vi "img test13(calibration attempt1).vi"() -> ()   [LabVIEW 2014]
uses:
  <vilib>/vision/NI_Vision_Development_Module.lvlib
panel:
  out "bottom player 2":cluster{"Numeric":dbl, "Numeric":dbl}[](array[cluster])
  out "bottom player":cluster{"Numeric":dbl, "Numeric":dbl}[](array[cluster])
  out "top player":cluster{"Numeric":dbl, "Numeric":dbl}[](array[cluster])
  out "size(s)":i32
  in  "playing":bool
  out "Top VIew":cluster{"Numeric":dbl, "Numeric":dbl}[](graph)
  out "Image 4":T1(plugin-control)
  in  "frame jump":i32=3
  in  "speed":u32(slide)=200
  in  "start":i32(slide) step=219843704 scale=0.0..263.0
  out "Image 3":T1(plugin-control)
  out "Image 2":T1(plugin-control)
  in  "AVI Path":path=path "C:/Users/Kokum Weeratunga/Desktop/img processing/ChenJin vs HuYun.avi"
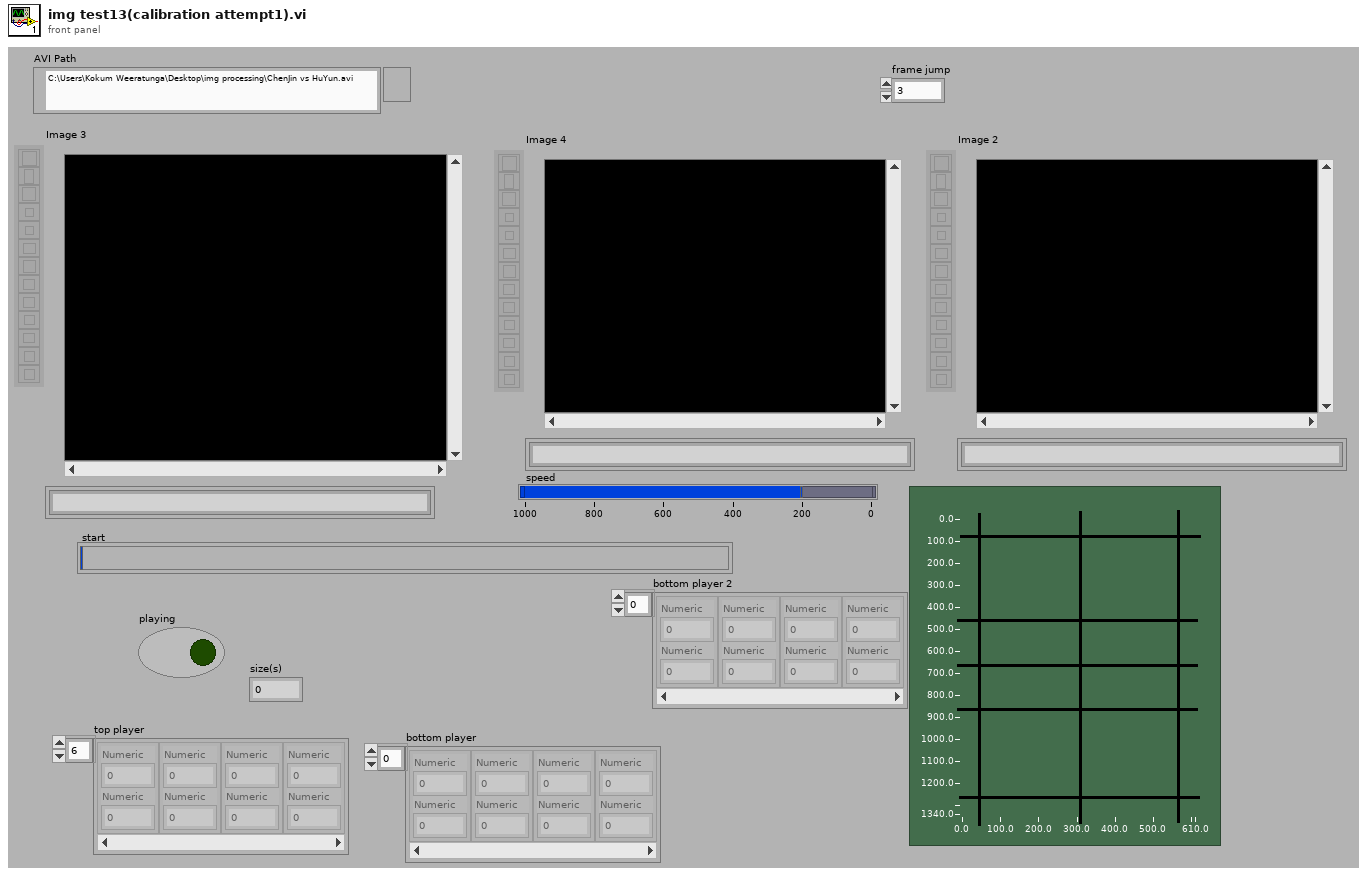
[diagram p1: front panel]
types:
  T1 = typedef "IMAQ Image.ctl" = refnum<image>
  T2 = typedef "Image Type" = u32
  T3 = typedef "AviRefnum.ctl" = refnum<k1>
  T4 = cluster{"width":u32, "height":u32, "framesPerSecond":u32, "compressionFilter":string, "hasData":bool}
  T5 = cluster{cluster{"X":sgl, "Y":sgl}[], cluster{i32, i32}[], "Unit":u32}
  T6 = cluster{"Origin Pixel":cluster{"X":sgl, "Y":sgl}, "Angle Relative to Horizontal (deg)":sgl, "Axis Reference":u32}
  T7 = typedef "Particle Parameters" = i32
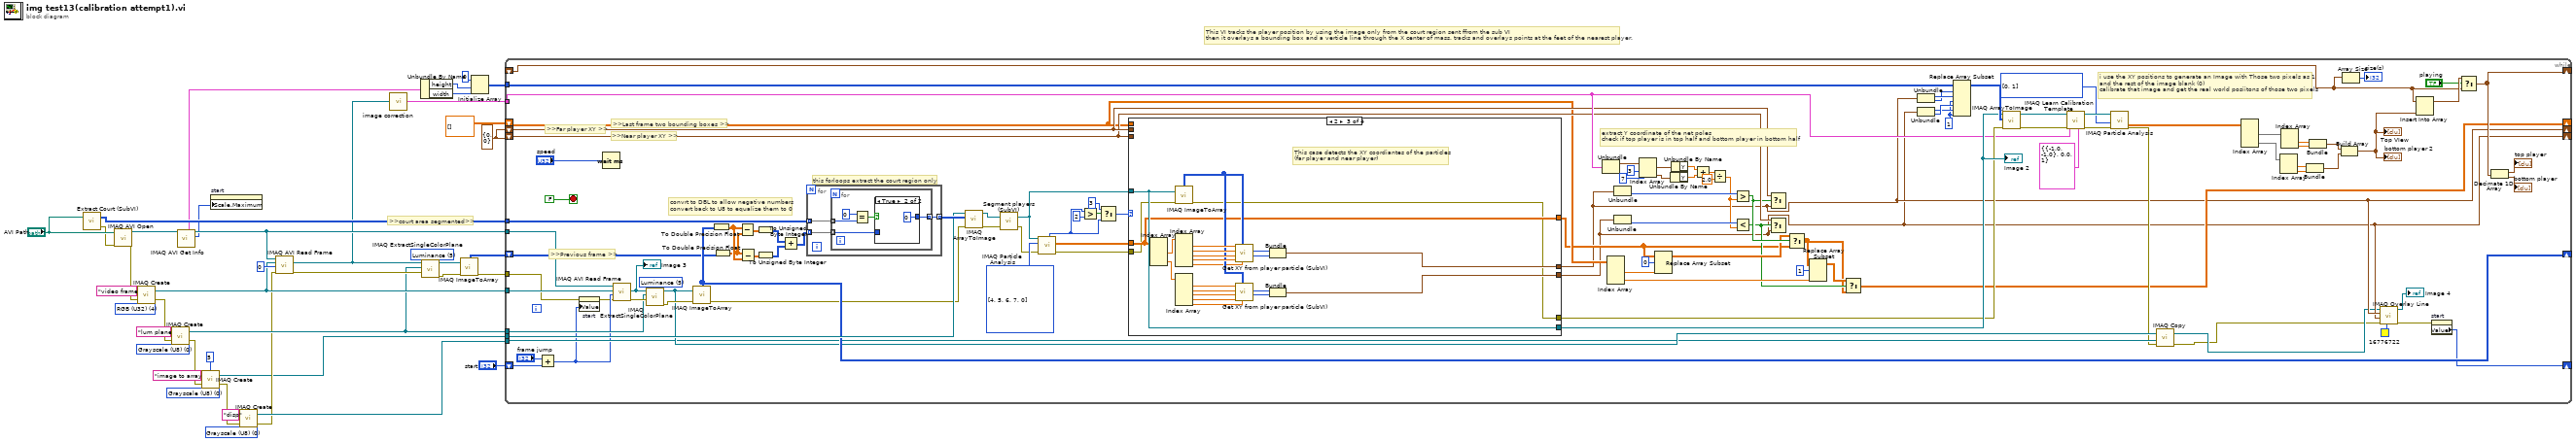
[diagram p0: block diagram]
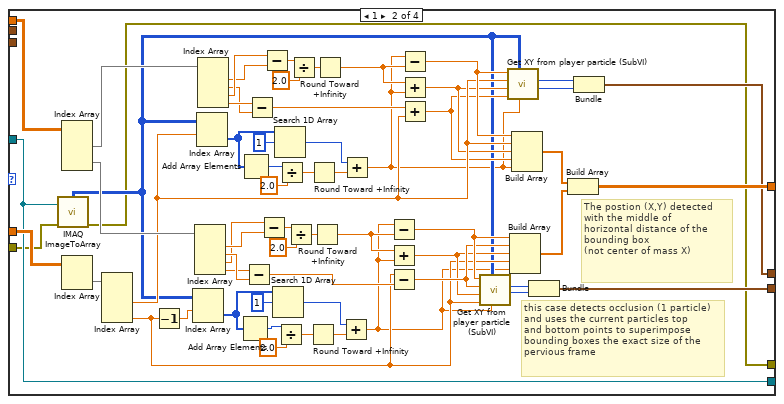
[diagram p3: hidden frame]
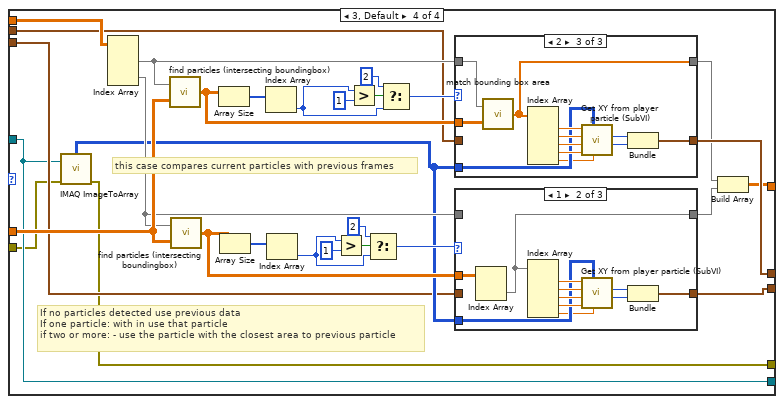
[diagram p4: hidden frame]
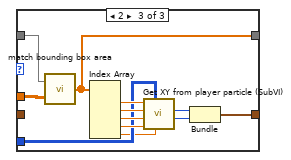
[diagram p6: hidden frame]
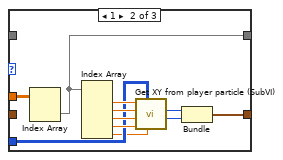
[diagram p8: hidden frame]
diagram:
  w13 = cluster{"X coordinate":i32, "Y coordinate":i32} {"X coordinate"=0, "Y coordinate"=0}
  w26 = T2 0 items=["Grayscale (U8)", "Grayscale (I16)", "Grayscale (SGL)", "Complex (CSG)", "RGB (U32)", "HSL (U32)", "RGB (U64)", "Grayscale (U16)"] ("Image Type")
  w33 = 5 items=["Red", "Green", "Blue", "Hue", "Saturation", "Luminance", "Value", "Intensity"] ("Color Plane")
  w34 = T2 0 items=["Grayscale (U8)", "Grayscale (I16)", "Grayscale (SGL)", "Complex (CSG)", "RGB (U32)", "HSL (U32)", "RGB (U64)", "Grayscale (U16)"] ("Image Type")
  w38 = T2 0 items=["Grayscale (U8)", "Grayscale (I16)", "Grayscale (SGL)", "Complex (CSG)", "RGB (U32)", "HSL (U32)", "RGB (U64)", "Grayscale (U16)"] ("Image Type")
  w36 = T2 4 items=["Grayscale (U8)", "Grayscale (I16)", "Grayscale (SGL)", "Complex (CSG)", "RGB (U32)", "HSL (U32)", "RGB (U64)", "Grayscale (U16)"] ("Image Type")
  # ">>court area segmented>>"
  # "This VI tracks the player position by using the image only from the court region sent ffrom the sub VI\nthen it overlays a bounding box and a verticle line through the X center of mass. tracks and overlays points at the feet of the nearest player."
  n1 = call "Extract Court (SubVI).vi"("AVI Path"="AVI Path") -> ("error out"=w40:errorcluster, "Court pixels out"=w16:u8[][])  [unwired: 1 in]
  n2 = call "IMAQ AVI Open"("error in (no error)"=w40, "AVI Path"="AVI Path") -> ("error out"=w22:errorcluster, "Avi Refnum"=w11:T3)  [unwired: 8 in]
  n3 = call "IMAQ Create"("Image Name"="video frame", "Image Type"=w36, "error in (no error)"=w22) -> ("New Image"=w30:T1, "error out"=w21:errorcluster)  [unwired: 2 in]
  n4 = call "IMAQ Create"("Image Name"="lum plane", "Image Type"=w38, "error in (no error)"=w21) -> ("New Image"=w29:T1, "error out"=w20:errorcluster)  [unwired: 2 in]
  n5 = call "IMAQ AVI Get Info"("Avi Refnum"=w11) -> ("Number of Frames"=w9:u32, "Avi Refnum (duplicate)"=w10:T3, "Frame Data"=w6:T4)  [unwired: 6 in, 2 out]
  n6 = call "IMAQ Create"("Border Size"=5, "Image Name"="image to array", "Image Type"=w34, "error in (no error)"=w20) -> ("New Image"=w15:T1, "error out"=w19:errorcluster)  [unwired: 1 in]
  n7 = property on="start" class="Slide (strict)"("Scale.Maximum"=w9) -> ()  [unwired: 2 in, 2 out]
  n8 = call "IMAQ Create"("Image Name"="disp", "Image Type"=w26, "error in (no error)"=w19) -> ("New Image"=w24:T1, "error out"=w18:errorcluster)  [unwired: 2 in]
  n9 = call "IMAQ AVI Read Frame"("error in (no error)"=w18, "Frame Number"=u32 0, "Image"=w30, "Avi Refnum"=w10) -> ("error out"=w32:errorcluster, "Image Out"=w2:T1)  [unwired: 4 in, 2 out]
  n10 = call "image correction.vi"("Image"=w2) -> ("ref points"=w1:T5)
  n11 = Unbundle By Name(w6) -> ("height"=w5:u32, "width"=w4:u32)
  n12 = call "IMAQ ExtractSingleColorPlane"("Color Plane"=w33, "error in (no error)"=w32, "Image Dst"=w29, "Image Src"=w2) -> ("error out"=w23:errorcluster, "Image Dst Out"=w27:T1)  [unwired: 6 in]
  n13 = call "IMAQ ImageToArray"("error in (no error)"=w23, "Image"=w27) -> ("error out"=w8:errorcluster, "Image Pixels (U8)"=w28:u8[][])  [unwired: 2 in, 3 out]
  n14 = Initialize Array(u8 0 ("element"), w5, w4) -> (w3:u8[][])
  n15 = while {
    tunnel: w10 -> [w111]
    tunnel: w30 -> [w131]
    tunnel: w16 -> [w148]
    tunnel: w29 -> [w132]
    tunnel: w15 -> [w145]
    shift-right: [w144] -> _
    shift-left: w28 -> [w143]
    tunnel: w24 -> [w114]
    shift-right: [w48] -> _
    shift-left: dbl[][] [] ("Particle Measurements (Pixels)") -> [w58]
    shift-right: [w46] -> _
    shift-left: w13 -> [w60]
    shift-right: [w45] -> _
    shift-left: w13 -> [w59]
    shift-right: [w106] -> _
    shift-left: "start" -> [w113]
    tunnel: w8 -> [w109]
    tunnel: w3 -> [w105]
    tunnel: w1 -> [w73]
    shift-right: [w76] -> _
    shift-left: _ -> [w80]
    stop <- FALSE stop-if-true
    w91 = T7[] [0, 1] items=["Center of Mass X", "Center of Mass Y", "First Pixel X", "First Pixel Y", "Bounding Rect Left", "Bounding Rect Top", "Bounding Rect Right", "Bounding Rect Bottom", "Max Feret Diameter Start X", "Max Feret Diameter Start Y", "Max Feret Diameter End X", "Max Feret Diameter End Y", "Max Horiz. Segment Length Left", "Max Horiz. Segment Length Right", "Max Horiz. Segment Length Row", "-", "Bounding Rect Width", "Bounding Rect Height", "Bounding Rect Diagonal", "Perimeter", "Convex Hull Perimeter", "Holes' Perimeter", "Max Feret Diameter", "Equivalent Ellipse Major Axis", "Equivalent Ellipse Minor Axis", "Equivalent Ellipse Minor Axis (Feret)", "Equivalent Rect Long Side", "Equivalent Rect Short Side", "Equivalent Rect Diagonal", "Equivalent Rect Short Side (Feret)", "Average Horiz. Segment Length", "Average Vert. Segment Length", "Hydraulic Radius", "Waddel Disk Diameter", "-", "Area", "Holes' Area", "Particle & Holes' Area", "Convex Hull Area", "Image Area", "-", "Number of Holes", "Number of Horiz. Segments", "Number of Vert. Segments", "-", "Orientation", "Max Feret Diameter Orientation", "-", "% Area/Image Area", "% Area/(Particle & Holes' Area)", "Ratio of Equivalent Ellipse Axes", "Ratio of Equivalent Rect Sides", "-", "Elongation Factor", "Compactness Factor", "Heywood Circularity Factor", "Type Factor", "-", "Sum X", "Sum Y", "Sum XX", "Sum XY", "Sum YY", "Sum XXX", "Sum XXY", "Sum XYY", "Sum YYY", "-", "Moment of Inertia XX", "Moment of Inertia XY", "Moment of Inertia YY", "Moment of Inertia XXX", "Moment of Inertia XXY", "Moment of Inertia XYY", "Moment of Inertia YYY", "Norm. Moment of Inertia XX", "Norm. Moment of Inertia XY", "Norm. Moment of Inertia YY", "Norm. Moment of Inertia XXX", "Norm. Moment of Inertia XXY", "Norm. Moment of Inertia XYY", "Norm. Moment of Inertia YYY", "Hu Moment 1", "Hu Moment 2", "Hu Moment 3", "Hu Moment 4", "Hu Moment 5", "Hu Moment 6", "Hu Moment 7"] ("Real-World Measurements")
    w100 = u8 1 ("new element/subarray")
    w133 = T7[] [4, 5, 6, 7, 0] items=["Center of Mass X", "Center of Mass Y", "First Pixel X", "First Pixel Y", "Bounding Rect Left", "Bounding Rect Top", "Bounding Rect Right", "Bounding Rect Bottom", "Max Feret Diameter Start X", "Max Feret Diameter Start Y", "Max Feret Diameter End X", "Max Feret Diameter End Y", "Max Horiz. Segment Length Left", "Max Horiz. Segment Length Right", "Max Horiz. Segment Length Row", "-", "Bounding Rect Width", "Bounding Rect Height", "Bounding Rect Diagonal", "Perimeter", "Convex Hull Perimeter", "Holes' Perimeter", "Max Feret Diameter", "Equivalent Ellipse Major Axis", "Equivalent Ellipse Minor Axis", "Equivalent Ellipse Minor Axis (Feret)", "Equivalent Rect Long Side", "Equivalent Rect Short Side", "Equivalent Rect Diagonal", "Equivalent Rect Short Side (Feret)", "Average Horiz. Segment Length", "Average Vert. Segment Length", "Hydraulic Radius", "Waddel Disk Diameter", "-", "Area", "Holes' Area", "Particle & Holes' Area", "Convex Hull Area", "Image Area", "-", "Number of Holes", "Number of Horiz. Segments", "Number of Vert. Segments", "-", "Orientation", "Max Feret Diameter Orientation", "-", "% Area/Image Area", "% Area/(Particle & Holes' Area)", "Ratio of Equivalent Ellipse Axes", "Ratio of Equivalent Rect Sides", "-", "Elongation Factor", "Compactness Factor", "Heywood Circularity Factor", "Type Factor", "-", "Sum X", "Sum Y", "Sum XX", "Sum XY", "Sum YY", "Sum XXX", "Sum XXY", "Sum XYY", "Sum YYY", "-", "Moment of Inertia XX", "Moment of Inertia XY", "Moment of Inertia YY", "Moment of Inertia XXX", "Moment of Inertia XXY", "Moment of Inertia XYY", "Moment of Inertia YYY", "Norm. Moment of Inertia XX", "Norm. Moment of Inertia XY", "Norm. Moment of Inertia YY", "Norm. Moment of Inertia XXX", "Norm. Moment of Inertia XXY", "Norm. Moment of Inertia XYY", "Norm. Moment of Inertia YYY", "Hu Moment 1", "Hu Moment 2", "Hu Moment 3", "Hu Moment 4", "Hu Moment 5", "Hu Moment 6", "Hu Moment 7"] ("Pixel Measurements")
    w149 = 5 items=["Red", "Green", "Blue", "Hue", "Saturation", "Luminance", "Value", "Intensity"] ("Color Plane")
    # "extract Y coordinate of the net poles\ncheck if top player is in top half and bottom player in bottom half"
    # "i use the XY positions to generate an Image with Those two pixels as 1 \nand the rest of the image blank (0)\ncalibrate that image and get the real world posiitons of those two pixels"
    # ">>Last frame two bounding boxes >>"
    # ">>Far player XY >>"
    # ">>Near player XY >>"
    # ">>Previous frame >>"
    # "convrt to DBL to allow negative numbers\nconvert back to U8 to equalize them to 0"
    # "this forloops extract the court region only"
    n16 = Add(x="frame jump", y=w113) -> (x+y=w110:i32)
    n17 = property on="start" class="Slide (strict)"(error in=w109, "Value"=w110) -> (error out=w108:errorcluster)  [unwired: 1 in, 1 out]
    n18 = Wait (ms)(milliseconds to wait="speed") -> ()  [unwired: 1 out]
    n19 = call "IMAQ AVI Read Frame"("error in (no error)"=w108, "Frame Number"=w110, "Image"=w131, "Avi Refnum"=w111) -> ("error out"=w150:errorcluster, "Image Out"=w128:T1)  [unwired: 4 in, 2 out]
    "Image 3" <- w128
    n20 = call "IMAQ ExtractSingleColorPlane"("Color Plane"=w149, "error in (no error)"=w150, "Image Dst"=w132, "Image Src"=w128) -> ("error out"=w135:errorcluster, "Image Dst Out"=w115:T1)  [unwired: 6 in]
    n21 = call "IMAQ ImageToArray"("error in (no error)"=w135, "Image"=w115) -> ("error out"=w134:errorcluster, "Image Pixels (U8)"=w144:u8[][])  [unwired: 2 in, 3 out]
    n22 = To Double Precision Float(number=w144) -> (double precision float=w139:dbl[][])
    n23 = To Double Precision Float(number=w143) -> (double precision float=w138:dbl[][])
    n24 = Subtract(x=w139, y=w138) -> (x-y=w137:dbl[][])
    n25 = Subtract(x=w138, y=w139) -> (x-y=w136:dbl[][])
    n26 = To Unsigned Byte Integer(number=w137) -> (unsigned 8bit integer=w142:u8[][])
    n27 = To Unsigned Byte Integer(number=w136) -> (unsigned 8bit integer=w141:u8[][])
    n28 = Add(x=w142, y=w141) -> (x+y=w140:u8[][])
    n29 = for {
      tunnel: w148 -> [w321] mode=indexing
      tunnel: [w320] -> w146 mode=indexing
      tunnel: w140 -> [w319] mode=indexing
      n30 = for {
        tunnel: w321 -> [w326] mode=indexing
        tunnel: [w323] -> w320 mode=indexing
        tunnel: w319 -> [w322] mode=indexing
        n31 = Equal?(x=u8 0, y=w326) -> (x = y?=w324:bool)
        n32 = case shown="True" w324 {
          tunnel: [w327 u8 0 ("x")] -> w323
          tunnel: w322 -> [w327 _]
          frame False {
          }
          frame True {
          }
        }
      }
    }
    n33 = call "IMAQ ArrayToImage"("error in (no error)"=w134, "Image Pixels (U8)"=w146, "Image"=w145) -> ("error out"=w129:errorcluster, "Image Out"=w130:T1)  [unwired: 7 in]
    n34 = call "Segment players (SubVI).vi"("error In"=w129, "Image In"=w130) -> ("error out"=w122:errorcluster, "Image Out"=w120:T1)
    n35 = call "IMAQ Particle Analysis"("error in (no error)"=w122, "Pixel Measurements"=w133, "Image"=w120) -> ("error out"=w121:errorcluster, "Particle Measurements (Pixels)"=w119:dbl[][], "Number of Particles"=w124:i32)  [unwired: 3 in, 3 out]
    n36 = Greater?(x=w124, y=2) -> (0:w127:bool)
    n37 = Select(t=3 ("y"), s=w127, f=w124) -> (s? t:f=w123:i32)
    n38 = case shown="2" w123 {
      tunnel: [w154 w181 w235 w245] -> w98
      tunnel: w119 -> [_ w216 w223 w265]
      tunnel: w121 -> [w151 w157 w220 w241]
      tunnel: w120 -> [w154 w181 w235 w245]
      tunnel: [w152 w165 w225 w247] -> w45
      tunnel: [w153 w172 w224 w246] -> w46
      tunnel: [w155 w182 w223 w242] -> w47
      tunnel: w58 -> [w155 w206 _ w268]
      tunnel: w60 -> [w153 _ _ w253]
      tunnel: w59 -> [w152 _ _ w248]
      tunnel: [w151 w156 w219 w240] -> w97
      frame 0 {
        # "This case identifies frames where no particles are detected and keeps the same values from the\nprevious frame"
      }
      frame 1 {
        # "The postion (X,Y) detected with the middle of \nhorizontal distance of the bounding box\n(not center of mass X)"
        # "this case detects occlusion (1 particle)\nand uses the current particles top \nand bottom points to superimpose \nbounding boxes the exact size of the \npervious frame"
        n39 = call "IMAQ ImageToArray"("error in (no error)"=w157, "Image"=w181) -> ("error out"=w156:errorcluster, "Image Pixels (U8)"=w164:u8[][])  [unwired: 2 in, 3 out]
        n40 = Index Array(array=w206) -> (element #1=w214:dbl[], element #2=w186:dbl[])  [unwired: 4 in]
        n41 = Index Array(array=w216) -> (element=w215:dbl[])  [unwired: 2 in]
        n42 = Index Array(array=w215) -> (element #2=w177:dbl, element #4=w168:dbl)  [unwired: 4 in, 2 out]
        n43 = Decrement(x=w168) -> (x-1=w179:dbl)
        n44 = Index Array(array=w164, index (row)=w179) -> (element=w201:u8[])  [unwired: 1 in]
        n45 = Index Array(array=w186) -> (element #1=w190:dbl, element #2=w193:dbl, element #3=w189:dbl, element #4=w192:dbl)  [unwired: 4 in]
        n46 = Index Array(array=w164, index (row)=w177) -> (element=w194:u8[])  [unwired: 1 in]
        n47 = Index Array(array=w214) -> (element #1=w210:dbl, element #2=w207:dbl, element #3=w211:dbl, element #4=w208:dbl)  [unwired: 4 in]
        n48 = Add Array Elements(numeric array=w201) -> (sum=w202:u8)
        n49 = Add Array Elements(numeric array=w194) -> (sum=w198:u8)
        n50 = Subtract(x=w192, y=w193) -> (x-y=w180:dbl)
        n51 = Subtract(x=w208, y=w207) -> (x-y=w185:dbl)
        n52 = Subtract(x=w189, y=w190) -> (x-y=w188:dbl)
        n53 = Subtract(x=w211, y=w210) -> (x-y=w212:dbl)
        n54 = Search 1D Array(1D array=w201, element=u8 1) -> (index of element=w200:i32)  [unwired: 1 in]
        n55 = Search 1D Array(1D array=w194, element=u8 1) -> (index of element=w199:i32)  [unwired: 1 in]
        n56 = Divide(x=w202, y=2.0) -> (x/y=w203:dbl)
        n57 = Divide(x=w198, y=2.0) -> (x/y=w197:dbl)
        n58 = Divide(x=w188, y=2.0) -> (x/y=w191:dbl)
        n59 = Divide(x=w212, y=2.0) -> (x/y=w209:dbl)
        n60 = Round Toward +Infinity(x=w203) -> (ceil(x): smallest int >= x=w162:dbl)
        n61 = Round Toward +Infinity(x=w197) -> (ceil(x): smallest int >= x=w161:dbl)
        n62 = Round Toward +Infinity(x=w191) -> (ceil(x): smallest int >= x=w163:dbl)
        n63 = Round Toward +Infinity(x=w209) -> (ceil(x): smallest int >= x=w160:dbl)
        n64 = Add(x=w200, y=w162) -> (x+y=w158:dbl)
        n65 = Add(x=w199, y=w161) -> (x+y=w159:dbl)
        n66 = Subtract(x=w158, y=w163) -> (x-y=w171:dbl)
        n67 = Add(x=w163, y=w158) -> (x+y=w169:dbl)
        n68 = Subtract(x=w168, y=w180) -> (x-y=w170:dbl)
        n69 = Subtract(x=w159, y=w160) -> (x-y=w178:dbl)
        n70 = Add(x=w160, y=w159) -> (x+y=w176:dbl)
        n71 = Add(x=w185, y=w177) -> (x+y=w175:dbl)
        n72 = call "Get XY from player particle (SubVI).vi"("Center of mass X"=w158, "Image in Pixels (U8)"=w164, "Particle bounding rect bottom"=w168, "Particle bounding rect right"=w169, "Particle bounding rect top"=w170, "Particle bounding rect left"=w171) -> ("Y coordinate"=w166:i32, "X coordinate"=w167:i32)  [unwired: 1 in, 1 out]
        n73 = call "Get XY from player particle (SubVI).vi"("Center of mass X"=w159, "Image in Pixels (U8)"=w164, "Particle bounding rect bottom"=w175, "Particle bounding rect right"=w176, "Particle bounding rect top"=w177, "Particle bounding rect left"=w178) -> ("Y coordinate"=w173:i32, "X coordinate"=w174:i32)  [unwired: 1 in, 1 out]
        n74 = Build Array(w171, w170, w169, w168, w158) -> (w183:dbl[])
        n75 = Build Array(w178, w177, w176, w175, w159) -> (w184:dbl[])
        n76 = Bundle("X coordinate"=w167, "Y coordinate"=w166) -> (w165:cluster{"X coordinate":i32, "Y coordinate":i32})  [unwired: 1 in]
        n77 = Build Array(w184, w183) -> (w182:dbl[][])
        n78 = Bundle("X coordinate"=w174, "Y coordinate"=w173) -> (w172:cluster{"X coordinate":i32, "Y coordinate":i32})  [unwired: 1 in]
      }
      frame 2 {
        # "This case detects the XY coordiantes of the particles\n(far player and near player)"
        n79 = Index Array(array=w223) -> (element #1=w229:dbl[], element #2=w228:dbl[])  [unwired: 4 in]
        n80 = call "IMAQ ImageToArray"("error in (no error)"=w220, "Image"=w235) -> ("error out"=w219:errorcluster, "Image Pixels (U8)"=w230:u8[][])  [unwired: 2 in, 3 out]
        n81 = Index Array(array=w229) -> (element #1=w239:dbl, element #2=w238:dbl, element #3=w237:dbl, element #4=w236:dbl, element #5=w222:dbl)  [unwired: 5 in]
        n82 = Index Array(array=w228) -> (element #1=w231:dbl, element #2=w232:dbl, element #3=w233:dbl, element #4=w234:dbl, element #5=w221:dbl)  [unwired: 5 in]
        n83 = call "Get XY from player particle (SubVI).vi"("Center of mass X"=w222, "Image in Pixels (U8)"=w230, "Particle bounding rect bottom"=w236, "Particle bounding rect right"=w237, "Particle bounding rect top"=w238, "Particle bounding rect left"=w239) -> ("Y coordinate"=w218:i32, "X coordinate"=w227:i32)  [unwired: 1 in, 1 out]
        n84 = call "Get XY from player particle (SubVI).vi"("Center of mass X"=w221, "Image in Pixels (U8)"=w230, "Particle bounding rect bottom"=w234, "Particle bounding rect right"=w233, "Particle bounding rect top"=w232, "Particle bounding rect left"=w231) -> ("Y coordinate"=w217:i32, "X coordinate"=w226:i32)  [unwired: 1 in, 1 out]
        n85 = Bundle("X coordinate"=w227, "Y coordinate"=w218) -> (w224:cluster{"X coordinate":i32, "Y coordinate":i32})  [unwired: 1 in]
        n86 = Bundle("X coordinate"=w226, "Y coordinate"=w217) -> (w225:cluster{"X coordinate":i32, "Y coordinate":i32})  [unwired: 1 in]
      }
      frame 3, Default {
        # "If no particles detected use previous data\nIf one particle: with in use that particle\nif two or more: - use the particle with the closest area to previous particle"
        # "this case compares current particles with previous frames"
        n87 = call "IMAQ ImageToArray"("error in (no error)"=w241, "Image"=w245) -> ("error out"=w240:errorcluster, "Image Pixels (U8)"=w249:u8[][])  [unwired: 2 in, 3 out]
        n88 = Index Array(array=w268) -> (element #1=w264:dbl[], element #2=w252:dbl[])  [unwired: 4 in]
        n89 = call "find particles (intersecting boundingbox).vi"("Particle Measurements in (bounding boxes)"=w265, "bounding box in"=w264) -> ("Particles within bounding box"=w263:dbl[][])
        n90 = call "find particles (intersecting boundingbox).vi"("Particle Measurements in (bounding boxes)"=w265, "bounding box in"=w252) -> ("Particles within bounding box"=w250:dbl[][])
        n91 = Array Size(array=w263) -> (size(s)=w267:i32[])
        n92 = Array Size(array=w250) -> (size(s)=w266:i32[])
        n93 = Index Array(array=w267) -> (element=w255:i32)  [unwired: 1 in]
        n94 = Index Array(array=w266) -> (element=w256:i32)  [unwired: 1 in]
        n95 = Greater?(x=w256, y=1) -> (0:w259:bool)
        n96 = Greater?(x=w255, y=1) -> (0:w260:bool)
        n97 = Select(t=2 ("y"), s=w259, f=w256) -> (s? t:f=w251:i32)
        n98 = Select(t=2 ("y"), s=w260, f=w255) -> (s? t:f=w254:i32)
        n99 = case shown="2" w254 {
          tunnel: w264 -> [w295 _ w310]
          tunnel: w263 -> [_ w306 w309]
          tunnel: [w295 w297 w308] -> w244
          tunnel: w249 -> [_ w299 w312]
          tunnel: [w294 w298 w311] -> w246
          tunnel: w253 -> [w294 _ _]
          frame 0, Default {
          }
          frame 1 {
            n100 = Index Array(array=w306) -> (element=w297:dbl[])  [unwired: 2 in]
            n101 = Index Array(array=w297) -> (element #1=w303:dbl, element #2=w302:dbl, element #3=w301:dbl, element #4=w300:dbl, element #5=w296:dbl)  [unwired: 5 in]
            n102 = call "Get XY from player particle (SubVI).vi"("Center of mass X"=w296, "Image in Pixels (U8)"=w299, "Particle bounding rect bottom"=w300, "Particle bounding rect right"=w301, "Particle bounding rect top"=w302, "Particle bounding rect left"=w303) -> ("Y coordinate"=w304:i32, "X coordinate"=w305:i32)  [unwired: 1 in, 1 out]
            n103 = Bundle("X coordinate"=w305, "Y coordinate"=w304) -> (w298:cluster{"X coordinate":i32, "Y coordinate":i32})  [unwired: 1 in]
          }
          frame 2 {
            n104 = call "match bounding box area.vi"("particle measurements (bounding box)"=w309, "bounding box in"=w310) -> ("matching bounding box"=w308:dbl[])
            n105 = Index Array(array=w308) -> (element #1=w316:dbl, element #2=w315:dbl, element #3=w314:dbl, element #4=w313:dbl, element #5=w307:dbl)  [unwired: 5 in]
            n106 = call "Get XY from player particle (SubVI).vi"("Center of mass X"=w307, "Image in Pixels (U8)"=w312, "Particle bounding rect bottom"=w313, "Particle bounding rect right"=w314, "Particle bounding rect top"=w315, "Particle bounding rect left"=w316) -> ("Y coordinate"=w317:i32, "X coordinate"=w318:i32)  [unwired: 1 in, 1 out]
            n107 = Bundle("X coordinate"=w318, "Y coordinate"=w317) -> (w311:cluster{"X coordinate":i32, "Y coordinate":i32})  [unwired: 1 in]
          }
        }
        n108 = case shown="1" w251 {
          tunnel: w252 -> [w270 _ w285]
          tunnel: w250 -> [_ w281 w284]
          tunnel: [w270 w272 w283] -> w243
          tunnel: w249 -> [_ w274 w287]
          tunnel: [w269 w273 w286] -> w247
          tunnel: w248 -> [w269 _ _]
          frame 0, Default {
          }
          frame 1 {
            n109 = Index Array(array=w281) -> (element=w272:dbl[])  [unwired: 2 in]
            n110 = Index Array(array=w272) -> (element #1=w278:dbl, element #2=w277:dbl, element #3=w276:dbl, element #4=w275:dbl, element #5=w271:dbl)  [unwired: 5 in]
            n111 = call "Get XY from player particle (SubVI).vi"("Center of mass X"=w271, "Image in Pixels (U8)"=w274, "Particle bounding rect bottom"=w275, "Particle bounding rect right"=w276, "Particle bounding rect top"=w277, "Particle bounding rect left"=w278) -> ("Y coordinate"=w279:i32, "X coordinate"=w280:i32)  [unwired: 1 in, 1 out]
            n112 = Bundle("X coordinate"=w280, "Y coordinate"=w279) -> (w273:cluster{"X coordinate":i32, "Y coordinate":i32})  [unwired: 1 in]
          }
          frame 2 {
            n113 = call "match bounding box area.vi"("particle measurements (bounding box)"=w284, "bounding box in"=w285) -> ("matching bounding box"=w283:dbl[])
            n114 = Index Array(array=w283) -> (element #1=w291:dbl, element #2=w290:dbl, element #3=w289:dbl, element #4=w288:dbl, element #5=w282:dbl)  [unwired: 5 in]
            n115 = call "Get XY from player particle (SubVI).vi"("Center of mass X"=w282, "Image in Pixels (U8)"=w287, "Particle bounding rect bottom"=w288, "Particle bounding rect right"=w289, "Particle bounding rect top"=w290, "Particle bounding rect left"=w291) -> ("Y coordinate"=w292:i32, "X coordinate"=w293:i32)  [unwired: 1 in, 1 out]
            n116 = Bundle("X coordinate"=w293, "Y coordinate"=w292) -> (w286:cluster{"X coordinate":i32, "Y coordinate":i32})  [unwired: 1 in]
          }
        }
        n117 = Build Array(w244, w243) -> (w242:dbl[][])
      }
    }
    "Image 2" <- w98
    n118 = Unbundle(w73) -> (w72:cluster{"X":sgl, "Y":sgl}[])  [unwired: 2 out]
    n119 = Index Array(array=w58) -> (element #1=w56:dbl[], element #2=w52:dbl[])  [unwired: 4 in]
    n120 = Unbundle(w45) -> ("Y coordinate"=w62:i32)  [unwired: 1 out]
    n121 = Unbundle(w46) -> ("Y coordinate"=w63:i32)  [unwired: 1 out]
    n122 = Index Array(array=w72, index #1=3 ("index"), index #2=7 ("index")) -> (element #1=w69:cluster{"X":sgl, "Y":sgl}, element #2=w68:cluster{"X":sgl, "Y":sgl})
    n123 = Replace Array Subset(array=w47, new element=w56, index (row)=0) -> (w55:dbl[][])  [unwired: 1 in]
    n124 = Unbundle By Name(w68) -> ("Y"=w66:sgl)
    n125 = Unbundle By Name(w69) -> ("Y"=w67:sgl)
    n126 = Add(x=w67, y=w66) -> (x+y=w65:sgl)
    n127 = Divide(x=w65, y=sgl 2.0) -> (x/y=w61:sgl)
    n128 = Greater?(x=w63, y=w61) -> (0:w57:bool)
    n129 = Less?(x=w62, y=w61) -> (x < y?=w50:bool)
    n130 = Select(t=w60, s=w57, f=w46) -> ()  [unwired: 1 out]
    n131 = Select(t=w59, s=w50, f=w45) -> ()  [unwired: 1 out]
    n132 = Select(t=w55, s=w57, f=w47) -> (s? t:f=w49:dbl[][])
    n133 = Replace Array Subset(array=w49, new element=w52, index (row)=1) -> (w51:dbl[][])  [unwired: 1 in]
    n134 = Select(t=w51, s=w50, f=w49) -> (s? t:f=w48:dbl[][])
    n135 = Unbundle(w45) -> ("X coordinate"=w101:i32, "Y coordinate"=w102:i32)
    n136 = Unbundle(w46) -> ("X coordinate"=w104:i32, "Y coordinate"=w103:i32)
    n137 = Replace Array Subset(array=w105, new element #1=w100, index (row) #1=w103, index (col) #1=w104, new element #2=w100, index (row) #2=w102, index (col) #2=w101) -> (w99:u8[][])
    n138 = call "IMAQ ArrayToImage"("error in (no error)"=w97, "Image Pixels (U8)"=w99, "Image"=w98) -> ("error out"=w94:errorcluster, "Image Out"=w95:T1)  [unwired: 7 in]
    n139 = call "IMAQ Learn Calibration Template"("Calibration Axis Info"=T6 {"Origin Pixel"={"X"=-1.0, "Y"=-1.0}, "Angle Relative to Horizontal (deg)"=0.0, "Axis Reference"=1}, "Reference Points"=w73, "error in (no error)"=w94, "Image"=w95) -> ("error out"=w93:errorcluster, "Calibrated Image"=w92:T1)  [unwired: 5 in, 1 out]
    n140 = call "IMAQ Particle Analysis"("error in (no error)"=w93, "Real-World Measurements"=w91, "Image"=w92) -> ("error out"=w90:errorcluster, "Particle Measurements (Real-World)"=w89:dbl[][])  [unwired: 3 in, 4 out]
    n141 = call "IMAQ Copy"("error in (no error)"=w90, "Image Dst"=w114, "Image Src"=w115) -> ("error out"=w42:errorcluster, "Image Dst Out"=w43:T1)  [unwired: 3 in]
    n142 = Index Array(array=w89) -> (element #1=w88:dbl[], element #2=w87:dbl[])  [unwired: 4 in]
    n143 = Index Array(array=w87) -> (element #1=w85:dbl, element #2=w86:dbl)  [unwired: 2 in]
    n144 = Index Array(array=w88) -> (element #1=w84:dbl, element #2=w83:dbl)  [unwired: 2 in]
    n145 = Bundle("Numeric"=w85, "Numeric"=w86) -> (w77:cluster{"Numeric":dbl, "Numeric":dbl})  [unwired: 1 in]
    n146 = Bundle("Numeric"=w84, "Numeric"=w83) -> (w78:cluster{"Numeric":dbl, "Numeric":dbl})  [unwired: 1 in]
    n147 = Build Array(w78, w77) -> (w44:cluster{"Numeric":dbl, "Numeric":dbl}[])
    "Top VIew" <- w44
    "bottom player 2" <- w44
    n148 = Array Size(array=w80) -> (size(s)=→"size(s)":i32)
    n149 = call "IMAQ Overlay Line"("Color"=u32 16776722, "error in (no error)"=w42, "End Point"=w45, "Start Point"=w46, "Image"=w43) -> ("error out"=w107:errorcluster, "Image Out"=→"Image 4":T1)  [unwired: 5 in]
    n150 = Insert Into Array(array=w80, new element=w44) -> (w82:cluster{"Numeric":dbl, "Numeric":dbl}[])  [unwired: 1 in]
    n151 = property on="start" class="Slide (strict)"(error in=w107) -> ("Value"=w106:i32)  [unwired: 1 in, 2 out]
    n152 = Select(t=w82, s="playing", f=w80) -> (s? t:f=w76:cluster{"Numeric":dbl, "Numeric":dbl}[])
    n153 = Decimate 1D Array(w76) -> (→"top player":cluster{"Numeric":dbl, "Numeric":dbl}[], →"bottom player":cluster{"Numeric":dbl, "Numeric":dbl}[])
  }
